vi "Waveform Generation - Process (8xI16).vi"(2 "Waveform Generation Resources":T1) -> ()   [LabVIEW 2018, in "Streaming FPGA.lvlib"]
doc: "Waveform Generation processing VI.\n\nConnect the <B>Waveform Generation Resources</B> input of this VI to the output of the <B>Waveform Generation - Create Resources.vi</B>."
uses:
  Streaming FPGA.lvlib
  Waveform Generation Resources (8xI16).ctl
  Target-Scoped FIFO (8xI16) Resource.ctl
  <vilib>/Platform/TimedLoop/XDataNode/timing_clust.ctl
  <vilib>/Platform/TimedLoop/XDataNode/nitl_modes.ctl
  <vilib>/Platform/TimedLoop/XDataNode/wakeup.ctl
  Data Storage - DRAM FIFO Priority.ctl
  <vilib>/rvi/Emulation/niFpgaSctlEmulationGetInTimedLoop.vi
  <vilib>/rvi/Emulation/niFpgaEmulationReportErrorSimple.vi
  <vilib>/rvi/Emulation/niFpgaGetClockAttributes.vi
  <vilib>/rvi/Emulation/niFpgaCriticalErrorInLSC.vi
  <vilib>/rvi/DataTransferAndStorage/Container/Common/niFpgaContainerExecOnDevCompGetState.vi
  <vilib>/rvi/Emulation/niFpgaEmulationIsFPGAContextNoSignature.vi
  <vilib>/rvi/DataTransferAndStorage/Container/Common/niFpgaContainerGetUniqueNameForEmu.vi
  <vilib>/rvi/Memory/Memory_Emulation/niFpgaMemoryEmulationCacheClearOnFirstRun.vi
  <vilib>/rvi/Memory/Memory_Emulation/nirvimemoryEmulationManagerCache_MakeExclusive.vi
  <vilib>/rvi/Memory/Memory_Emulation/niFpgaMemoryEmulationValidateCache.vi
  <vilib>/rvi/Memory/Memory_Emulation/nirvimemoryEmulationManagerCache_InsertValue.vi
  <vilib>/Utility/error.llb/Clear Errors.vi
  <vilib>/rvi/Memory/Memory_Emulation/nirvimemoryEmulationManagerCache_ReleaseExclusive.vi
  <vilib>/rvi/Memory/Memory_Emulation/nirvimemoryEmulationManagerCache_GetValue.vi
  <vilib>/rvi/Memory/Memory_Emulation/nirvimemoryEmulationManagerCache_SetValue.vi
  <vilib>/rvi/Emulation/niFpgaProcessEmulError.vi
  <vilib>/rvi/errors/niFpgaSetErrorForExecOnDevCompSimple.vi
  <vilib>/rvi/eio/common/nirviEmuReportErrorAndStop.vi
  <vilib>/rvi/interface/RandomDataEmulation/nirviRandomDataAcquireLock.vi
  <vilib>/rvi/interface/RandomDataEmulation/nirviRandomDataQueueStore.vi
  <vilib>/rvi/interface/RandomDataEmulation/nirviRandomDataReleaseLock.vi
  <vilib>/rvi/interface/RandomDataEmulation/nirviFPGAContextMergeError.vi
  <vilib>/rvi/interface/RandomDataEmulation/nirviRandomDataCheckExitLoopConditions.vi
  <vilib>/express/rvi/timingcommon/nirviCommon.vi
  <vilib>/rvi/interface/RandomDataEmulation/niFpgaRandomDataHandleErrors.vi
  <instrlib>/_niInstr/Basic Elements/v1/FPGA/Private/Count Up U32.vi
  <vilib>/platform/TimedLoop/XDataNode/XDataNode.xnode
  <vilib>/rvi/DataTransferAndStorage/Container/XNode/niFpgaContainer.xnode
  <vilib>/rvi/DataTransferAndStorage/Register/Emulation/niFpgaRegisterEmulationRefIn.vi
  <vilib>/rvi/FIFO/Fifo_Resource/niFpgaFifoEmulationRefInMultiElement.vi
  <vilib>/Platform/TimedLoop/XDataNode/XDNodeRunTimeDep.lvlib
  <instrlib>/_niInstr/Basic Elements/v1/FPGA/niInstr Basic Elements v1 FPGA.lvlib
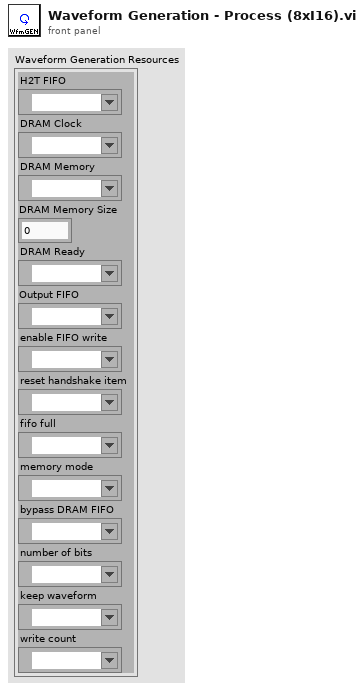
[diagram p1: front panel]
types:
  T1 = typedef "Streaming FPGA.lvlib/Waveform Generation Resources (8xI16).ctl" = cluster{"H2T FIFO":refnum<k21>, "DRAM Clock":refnum<k21>, "DRAM Memory":refnum<k21>, "DRAM Memory Size":u32, "DRAM Ready":refnum<k21>, "Output FIFO":T2, "enable FIFO write":refnum<k21>, "reset handshake item":refnum<k21>, "fifo full":refnum<k21>, "memory mode":refnum<k21>, "bypass DRAM FIFO":refnum<k21>, "number of bits":refnum<k21>, "keep waveform":refnum<k21>, "write count":refnum<k21>}
  T2 = typedef "Streaming FPGA.lvlib/Target-Scoped FIFO (8xI16) Resource.ctl" = refnum<k21>
  T3 = typedef "XDNodeRunTimeDep.lvlib/timing_clust.ctl" = cluster{"Expected End [f-1]":u64, "Actual End [f-1]":u64, "Finished Late? [f-1]":bool, "Expected End [i-1]":u64, "Actual End [i-1]":u64, "Finished Late? [i-1]":bool, "Expected Start [i]":u64, "Actual Start [i]":u64, "Expected Start [f]":u64, "Actual Start [f]":u64, "Source Name":string, "Structure Name":string, "Period":i64, "Deadline":i64, "Offset":i64, "Start":i64, "Priority":i32, "Timeout":i32, "Mode":T4, "Wakeup Reason":T5, "Error":errorcluster, "Source Type":string, "Secondary Source Type":string, "Global End Time":u64, "Global Start Time":u64, "Frame Duration":u64, "Iteration Duration":u64, "Assigned CPU":i32, "I/O Scan Engine Mode":u32}
  T4 = typedef "XDNodeRunTimeDep.lvlib/nitl_modes.ctl" = enum32{"No Change", "Process missed periods, maintain original phase", "Discard missed periods, maintain original phase", "Process missed periods, ignore original phase", "Discard missed periods, ignore original phase"}
  T5 = typedef "XDNodeRunTimeDep.lvlib/wakeup.ctl" = enum32{"Normal", "Aborted", "Asynchronous wakeup", "Timing source error", "Timed loop error", "Timeout"}
  T6 = typedef "Streaming FPGA.lvlib/Data Storage - DRAM FIFO Priority.ctl" = enum16{"balanced", "favor writes", "favor reads"}
  T7 = typedef "Streaming FPGA.lvlib/Data Type (16xI16).ctl" = i16[]
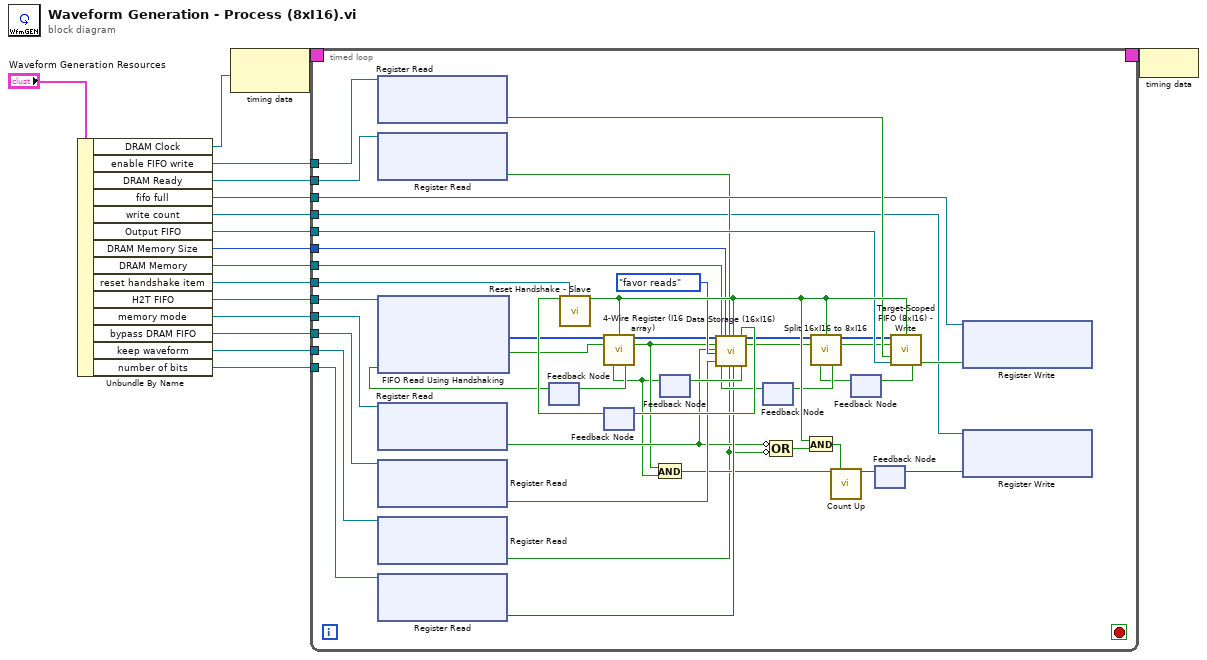
[diagram p0: block diagram]
diagram:
  n1 = Unbundle By Name("Waveform Generation Resources") -> ("DRAM Clock"=w2:refnum<k21>, "enable FIFO write"=w1:refnum<k21>, "DRAM Ready"=w8:refnum<k21>, "fifo full"=w11:refnum<k21>, "write count"=w3:refnum<k21>, "Output FIFO"=w16:T2, "DRAM Memory Size"=w6:u32, "DRAM Memory"=w17:refnum<k21>, "reset handshake item"=w13:refnum<k21>, "H2T FIFO"=w14:refnum<k21>, "memory mode"=w12:refnum<k21>, "bypass DRAM FIFO"=w7:refnum<k21>, "keep waveform"=w5:refnum<k21>, "number of bits"=w4:refnum<k21>)
  n2 = node-c288(w2) -> (w10:T3)
  n3 = timed-loop {
    timing: w10 -> [_]
    timing-out: [_] -> w9
    tunnel: w17 -> [w42]
    tunnel: w16 -> [w58]
    tunnel: w14 -> [w52]
    tunnel: w13 -> [w51]
    tunnel: w12 -> [w50]
    tunnel: w11 -> [w49]
    tunnel: w8 -> [w47]
    tunnel: w7 -> [w46]
    tunnel: w6 -> [w34]
    tunnel: w5 -> [w32]
    tunnel: w4 -> [w31]
    tunnel: w3 -> [w27]
    tunnel: w1 -> [w21]
    stop <- _ stop-if-true
    n4 = xnode "Register Read"("Register In"=w21) -> ("Data"=w61:bool)  [unwired: 1 out]
    n5 = xnode "Register Read"("Register In"=w47) -> ("Data"=w41:bool)  [unwired: 1 out]
    n6 = xnode "Register Read"("Register In"=w50) -> ("Data"=w25:bool)  [unwired: 1 out]
    n7 = xnode "Register Read"("Register In"=w46) -> ("Data"=w33:bool)  [unwired: 1 out]
    n8 = xnode "Register Read"("Register In"=w32) -> ("Data"=w24:bool)  [unwired: 1 out]
    n9 = xnode "Register Read"("Register In"=w31) -> ("Data"=w30:u64)  [unwired: 1 out]
    n10 = feedback #1() -> (w54:bool)  [unwired: 1 in]
    n11 = xnode "FIFO Read Using Handshaking"("Ready for Output"=w54, "FIFO In"=w52) -> ("Element"=w57:i16[], "Output Valid"=w56:bool)  [unwired: 1 out]
    n12 = feedback #2() -> (w59:bool)  [unwired: 1 in]
    n13 = call "Reset Handshake - Slave.vi"("reset done"=w59, "reset handshake item"=w51) -> ("reset"=w62:bool)  [unwired: 13 in]
    n14 = feedback #3() -> (w18:bool)  [unwired: 1 in]
    n15 = call "4-Wire Register (I16 array).vi"("data in"=w57, "reset"=w62, "input valid"=w56, "ready for output (T)"=w18) -> ("data out"=w20:i16[], "output valid"=w19:bool, "ready for input"=w55:bool)  [unwired: 9 in]
    n16 = feedback-in #1(w55) -> ()
    n17 = And(x=w19, y=w18) -> (x .and. y?=w29:bool)
    n18 = feedback #4() -> (w40:bool)  [unwired: 1 in]
    n19 = call "Data Storage (16xI16).vi"("data in"=w20, "input valid"=w19, "memory mode (F)"=w25, "priority (balanced)"=Data_Storage_-_DRAM_FIFO_Priority."favor reads", "bypass DRAM FIFO (F)"=w33, "DRAM Memory"=w42, "ready for output (T)"=w40, "Memory Size"=w34, "DRAM Ready"=w41, "keep data (F)"=w24, "reset"=w62, "# of bits"=w30) -> ("reset done"=w43:bool, "ready for input"=w44:bool, "data out"=w39:T7, "output valid"=w38:bool)  [unwired: 12 in]
    n20 = feedback-in #2(w43) -> ()
    n21 = feedback-in #3(w44) -> ()
    n22 = Compound Arithmetic op=OR(invert w25, invert w24) -> (w23:bool)
    n23 = And(x=w62, y=w23) -> (x .and. y?=w22:bool)
    n24 = call-poly <instrlib>:"Count Up.vi"("increment"=w29, "reset"=w22) -> ("count out"=w28:u32)  [unwired: 13 in]
    n25 = feedback #5() -> (w35:bool)  [unwired: 1 in]
    n26 = call "Split 16xI16 to 8xI16.vi"("data in"=w39, "reset"=w62, "input valid"=w38, "ready for output (T)"=w35) -> ("data out"=w37:i16[], "output valid"=w36:bool, "ready for input"=w53:bool)  [unwired: 9 in]
    n27 = feedback-in #4(w53) -> ()
    n28 = feedback-in #6(w28) -> ()
    n29 = feedback #6() -> (w26:u32)  [unwired: 1 in]
    n30 = call "Target-Scoped FIFO (8xI16) - Write.vi"("data in"=w37, "reset"=w62, "input valid"=w36, "write enable (T)"=w61, "Target-Scoped FIFO (8xI16)"=w58) -> ("ready for input"=w45:bool, "fifo full"=w48:bool)  [unwired: 9 in]
    n31 = feedback-in #5(w45) -> ()
    n32 = xnode "Register Write"("Data"=w48, "Register In"=w49) -> ()  [unwired: 1 out]
    n33 = xnode "Register Write"("Data"=w26, "Register In"=w27) -> ()  [unwired: 1 out]
  }
  n34 = node-c288(w9) -> ()
